vi "Perform Auto-Click.vi"(7 "No Oxy?":bool, 8 "error in (no error)":errorcluster, 9 "Monitor Resolutions":cluster{"V":i16, "H":i16}[](array[cluster]), 10 "Monitor":i32, 11 "Levels":T1) -> (0 "error out":errorcluster)   [LabVIEW 2021]
uses:
  0d922631-5a7c-4ace-b290-72c775d65e45.vi
  ab490d8f-ff69-4fb2-997c-3fcb65ef86d5.vi
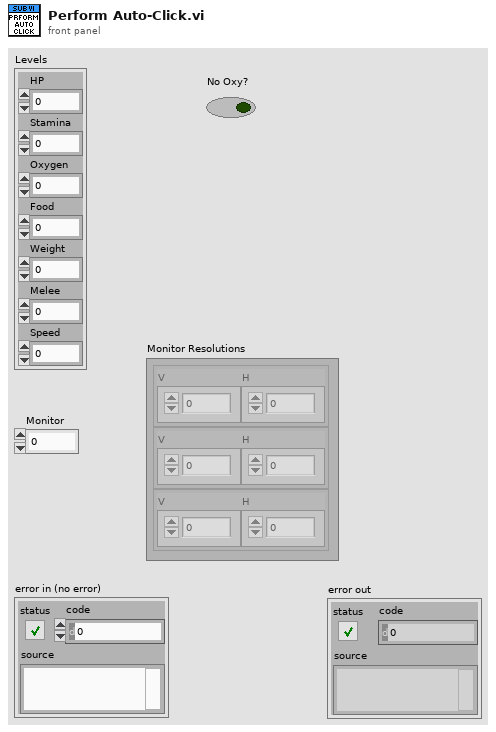
[diagram p1: front panel]
types:
  T1 = cluster{"HP":i32, "Stamina":i32, "Oxygen":i32, "Food":i32, "Weight":i32, "Melee":i32, "Speed":i32}
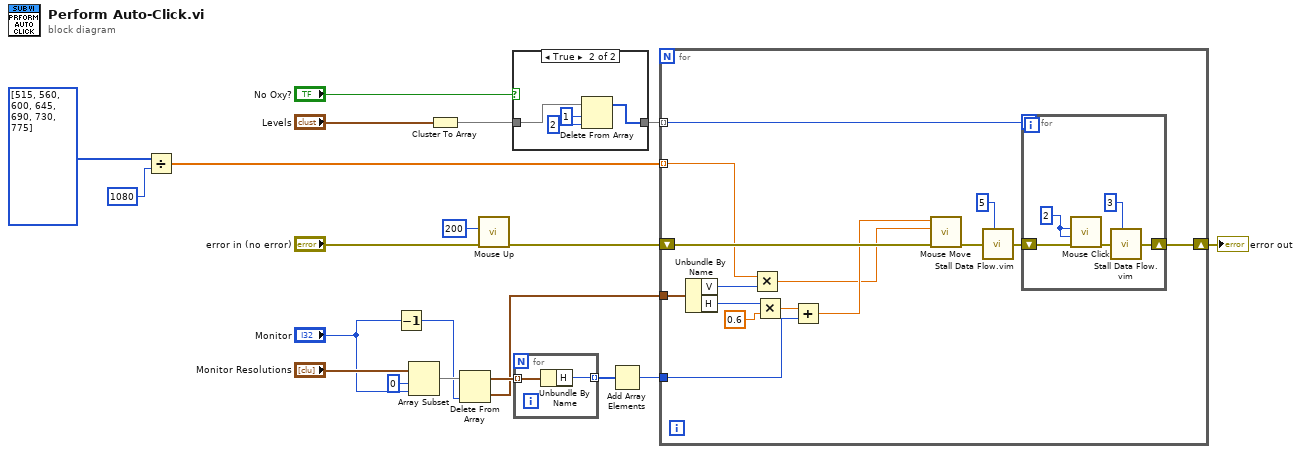
[diagram p0: block diagram]
diagram:
  n1 = Divide(x=i32[] [515, 560, 600, 645, 690, 730, 775], y=1080) -> (x/y=w4:dbl[])
  n2 = Decrement(x="Monitor") -> (x-1=w11:i32)
  n3 = Array Subset(array="Monitor Resolutions", index=0, length="Monitor") -> (w13:cluster{"V":i16, "H":i16}[])
  n4 = Cluster To Array(cluster="Levels") -> (array=w18:i32[])
  n5 = Delete From Array(array=w13, index=w11) -> (deleted portion=w8:cluster{"V":i16, "H":i16}, array with subset deleted=w10:cluster{"V":i16, "H":i16}[])  [unwired: 1 in]
  n6 = call "Mouse Up.vi"("error in (no error)"="error in (no error)", "Delay in ms (10)"=u32 200 ("milliseconds to wait")) -> ("error out"=w3:errorcluster)  [unwired: 9 in]
  n7 = case shown="True" "No Oxy?" {
    tunnel: w18 -> [w21 w25]
    tunnel: [w21 w22] -> w17
    frame False {
    }
    frame True {
      n8 = Delete From Array(array=w25, length=1, index=2) -> (array with subset deleted=w22:i32[])  [unwired: 1 out]
    }
  }
  n9 = for {
    tunnel: w10 -> [w27] mode=indexing
    tunnel: [w26] -> w9 mode=indexing
    n10 = Unbundle By Name(w27) -> ("H"=w26:i16)
  }
  n11 = Add Array Elements(numeric array=w9) -> (sum=w7:i16)
  n12 = for {
    tunnel: w17 -> [w41] mode=indexing
    tunnel: w4 -> [w30] mode=indexing
    shift-right: [w40] -> w19
    shift-left: w3 -> [w42]
    tunnel: w8 -> [w36]
    tunnel: w7 -> [w32]
    n13 = Unbundle By Name(w36) -> ("V"=w31:i16, "H"=w34:i16)
    n14 = Multiply(x=w30, y=w31) -> (x*y=w28:dbl)
    n15 = Multiply(x=w34, y=0.6) -> (x*y=w33:dbl)
    n16 = Add(x=w33, y=w32) -> (x+y=w29:dbl)
    n17 = call "Mouse Move.vi"("error in (no error)"=w42, "y"=w28, "x"=w29) -> ("error out"=w38:errorcluster)  [unwired: 8 in]
    n18 = call "Stall Data Flow.vim"("value in"=w38, "milliseconds to wait"=u32 5) -> ("value out"=w37:errorcluster)  [unwired: 1 out]
    n19 = for {
      N: w41 -> [_]
      shift-right: [w45] -> w40
      shift-left: w37 -> [w47]
      w43 = u32 2 ("ms wait after down (10)")
      n20 = call "Mouse Click.vi"("error in (no error)"=w47, "ms wait after up (10)"=w43, "ms wait after down (10)"=w43) -> ("error out"=w46:errorcluster)  [unwired: 8 in]
      n21 = call "Stall Data Flow.vim"("value in"=w46, "milliseconds to wait"=u32 3) -> ("value out"=w45:errorcluster)  [unwired: 1 out]
    }
  }
  "error out" <- w19
